vi "Read Request Key to Value.vi"(10 "Request Keys":T2, 11 "Request":T1={"Key"=["SERVER_PROTOCOL", "SERVER_SOFTWARE", "GATEWAY_INTERFACE", "SERVER_PORT", "SERVER_NAME", "DOCUMENT_ROOT", "SERVER_URL", "SERVER_ADDR", "SERVER_HOST", "QUERY_STRING", "CONTENT_LENGTH", "PATH_INFO", "SCRIPT_FILENAME", "AUTH_TYPE", "REMOTE_HOST", "SERVICE_NAME", "REQUEST_URI", "SERVICE_PATH", "REQUEST_TRANSPORT", "SCRIPT_NAME", "CONTENT_TYPE", "PATH_TRANSLATED", "REMOTE_USER", "REMOTE_ADDR", "REQUEST_METHOD", "CONTENT_LENGTH", "HOST", "CONNECTION", "REFERER", "ACCEPT", "CACHE_CONTROL", "ACCEPT_ENCODING", "CONTENT_TYPE", "ACCEPT_CHARSET", "ACCEPT_LANGUAGE", "USER_AGENT", "ORIGIN", "ProjectCity", "Language", "Q.Plant0.001", "ProjectTitle", "Email", "Name", "countries", "Organization", "ProjectNotes", "ProjectState"], "Value"=[]}) -> (3 "Value":string)   [LabVIEW 2015]
uses:
  RequestKeys.ctl
  user project design.ctl
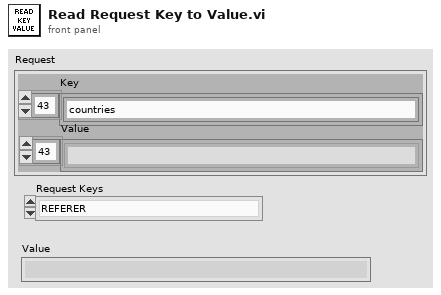
[diagram p1: front panel]
types:
  T1 = typedef "user project design.ctl" = cluster{"Key":string[], "Value":string[]}
  T2 = typedef "RequestKeys.ctl" = enum16{"REFERER", "Name", "Email", "Organization", "Language", "Country", "ProjectTitle", "ProjectCity", "ProjectState", "ProjectNotes"}
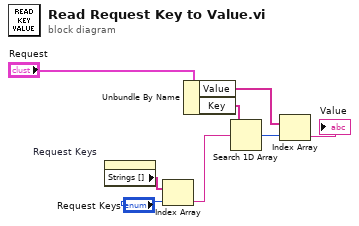
[diagram p0: block diagram]
diagram:
  n1 = property on="Request Keys" class="Enum (strict)"() -> ("Strings []"=w8:string[])  [unwired: 2 in, 2 out]
  n2 = Index Array(array=w8, index="Request Keys") -> (element=w6:string)
  n3 = Unbundle By Name("Request") -> ("Value"=w2:string[], "Key"=w4:string[])
  n4 = Search 1D Array(1D array=w4, element=w6) -> (index of element=w3:i32)  [unwired: 1 in]
  n5 = Index Array(array=w2, index=w3) -> (element=→"Value":string)
